vi "nanocal -- nuclear schottky fit V4.vi"() -> ()   [LabVIEW 2020] (continued)
RAW_cal__ref_"="IDS0317_210901_RAW_cal_CeCoIn5_4th_046(132)_C(f)_12T_0.43K_45deg_Tdep_raw_.dat", "IDS0317_210901_RAW_cal__sam_"="IDS0317_210901_RAW_cal_CeCoIn5_4th_046(132)_C(f)_12T_0.43K_45deg_Tdep_raw_.dat", "IDS0318_210901_RAW_cal__ref_"="IDS0318_210901_RAW_cal_CeCoIn5_4th_047(133)_C(f)_12T_0.53K_45deg_Tdep_raw_.dat", "IDS0318_210901_RAW_cal__sam_"="IDS0318_210901_RAW_cal_CeCoIn5_4th_047(133)_C(f)_12T_0.53K_45deg_Tdep_raw_.dat", "IDS0319_210901_RAW_cal__ref_"="IDS0319_210901_RAW_cal_CeCoIn5_4th_048(134)_C(f)_12T_0.62K_45deg_Tdep_raw_.dat", "IDS0319_210901_RAW_cal__sam_"="IDS0319_210901_RAW_cal_CeCoIn5_4th_048(134)_C(f)_12T_0.62K_45deg_Tdep_raw_.dat", "IDS0320_210901_RAW_cal__ref_"="IDS0320_210901_RAW_cal_CeCoIn5_4th_049(135)_C(f)_12T_0.83K_45deg_Tdep_raw_.dat", "IDS0320_210901_RAW_cal__sam_"="IDS0320_210901_RAW_cal_CeCoIn5_4th_049(135)_C(f)_12T_0.83K_45deg_Tdep_raw_.dat", "IDS0321_210901_RAW_cal__ref_"="IDS0321_210901_RAW_cal_CeCoIn5_4th_050(136)_C(f)_12T_1.13K_45deg_Tdep_raw_.dat", "IDS0321_210901_RAW_cal__sam_"="IDS0321_210901_RAW_cal_CeCoIn5_4th_050(136)_C(f)_12T_1.13K_45deg_Tdep_raw_.dat", "IDS0322_210901_RAW_cal__ref_"="IDS0322_210901_RAW_cal_CeCoIn5_4th_051(137)_C(f)_12T_1.90K_45deg_Tdep_raw_.dat", "IDS0322_210901_RAW_cal__sam_"="IDS0322_210901_RAW_cal_CeCoIn5_4th_051(137)_C(f)_12T_1.90K_45deg_Tdep_raw_.dat", "IDS0323_210901_RAW_cal__ref_"="IDS0323_210901_RAW_cal_CeCoIn5_4th_052(138)_C(f)_12T_3.10K_45deg_Tdep_raw_.dat", "IDS0323_210901_RAW_cal__sam_"="IDS0323_210901_RAW_cal_CeCoIn5_4th_052(138)_C(f)_12T_3.10K_45deg_Tdep_raw_.dat", "IDS0324_210901_RAW_cal__ref_"="IDS0324_210901_RAW_cal_CeCoIn5_4th_053(139)_C(f)_12T_5.70K_45deg_Tdep_raw_.dat", "IDS0324_210901_RAW_cal__sam_"="IDS0324_210901_RAW_cal_CeCoIn5_4th_053(139)_C(f)_12T_5.70K_45deg_Tdep_raw_.dat", "IDS0330_210901_RAW_cal__ref_"="IDS0330_210901_RAW_cal_CeCoIn5_4th_059_C(f)_1T_0.197K_90deg_Bdep_raw_.dat", "IDS0330_210901_RAW_cal__sam_"="IDS0330_210901_RAW_cal_CeCoIn5_4th_059_C(f)_1T_0.197K_90deg_Bdep_raw_.dat", "IDS0331_210901_RAW_cal__ref_"="IDS0331_210901_RAW_cal_CeCoIn5_4th_060_C(f)_2T_0.197K_90deg_Bdep_raw_.dat", "IDS0331_210901_RAW_cal__sam_"="IDS0331_210901_RAW_cal_CeCoIn5_4th_060_C(f)_2T_0.197K_90deg_Bdep_raw_.dat", "IDS0335_210904_RAW_cal__ref_"="IDS0335_210904_RAW_cal_CeCoIn5_4th_064_C(f)_5.0T_0.197K_90deg_fsweep_Tdep_raw_.dat", "IDS0335_210904_RAW_cal__sam_"="IDS0335_210904_RAW_cal_CeCoIn5_4th_064_C(f)_5.0T_0.197K_90deg_fsweep_Tdep_raw_.dat", "IDS0336_210904_RAW_cal__ref_"="IDS0336_210904_RAW_cal_CeCoIn5_4th_065_C(f)_5.0T_0.122K_90deg_fsweep_Tdep_raw_.dat", "IDS0336_210904_RAW_cal__sam_"="IDS0336_210904_RAW_cal_CeCoIn5_4th_065_C(f)_5.0T_0.122K_90deg_fsweep_Tdep_raw_.dat", "IDS0337_210904_RAW_cal__ref_"="IDS0337_210904_RAW_cal_CeCoIn5_4th_066_C(f)_5.0T_0.157K_90deg_Tdep_raw_.dat", "IDS0337_210904_RAW_cal__sam_"="IDS0337_210904_RAW_cal_CeCoIn5_4th_066_C(f)_5.0T_0.157K_90deg_Tdep_raw_.dat", "IDS0338_210904_RAW_cal__ref_"="IDS0338_210904_RAW_cal_CeCoIn5_4th_067_C(f)_5.0T_0.170K_90deg_Tdep_raw_.dat", "IDS0338_210904_RAW_cal__sam_"="IDS0338_210904_RAW_cal_CeCoIn5_4th_067_C(f)_5.0T_0.170K_90deg_Tdep_raw_.dat", "IDS0339_210904_RAW_cal__ref_"="IDS0339_210904_RAW_cal_CeCoIn5_4th_068_C(f)_5.0T_0.255K_90deg_Tdep_raw_.dat", "IDS0339_210904_RAW_cal__sam_"="IDS0339_210904_RAW_cal_CeCoIn5_4th_068_C(f)_5.0T_0.255K_90deg_Tdep_raw_.dat", "IDS0340_210904_RAW_cal__ref_"="IDS0340_210904_RAW_cal_CeCoIn5_4th_069_C(f)_5.0T_0.308K_90deg_Tdep_raw_.dat", "IDS0340_210904_RAW_cal__sam_"="IDS0340_210904_RAW_cal_CeCoIn5_4th_069_C(f)_5.0T_0.308K_90deg_Tdep_raw_.dat", "IDS0341_210904_RAW_cal__ref_"="IDS0341_210904_RAW_cal_CeCoIn5_4th_070_C(f)_5.0T_0.360K_90deg_Tdep_raw_.dat", "IDS0341_210904_RAW_cal__sam_"="IDS0341_210904_RAW_cal_CeCoIn5_4th_070_C(f)_5.0T_0.360K_90deg_Tdep_raw_.dat", "IDS0342_210904_RAW_cal__ref_"="IDS0342_210904_RAW_cal_CeCoIn5_4th_071_C(f)_5.0T_0.438K_90deg_Tdep_raw_.dat", "IDS0342_210904_RAW_cal__sam_"="IDS0342_210904_RAW_cal_CeCoIn5_4th_071_C(f)_5.0T_0.438K_90deg_Tdep_raw_.dat", "IDS0343_210904_RAW_cal__ref_"="IDS0343_210904_RAW_cal_CeCoIn5_4th_072_C(f)_5.0T_0.53K_90deg_Tdep_raw_.dat", "IDS0343_210904_RAW_cal__sam_"="IDS0343_210904_RAW_cal_CeCoIn5_4th_072_C(f)_5.0T_0.53K_90deg_Tdep_raw_.dat", "IDS0344_210904_RAW_cal__ref_"="IDS0344_210904_RAW_cal_CeCoIn5_4th_073_C(f)_5.0T_0.62K_90deg_Tdep_raw_.dat", "IDS0344_210904_RAW_cal__sam_"="IDS0344_210904_RAW_cal_CeCoIn5_4th_073_C(f)_5.0T_0.62K_90deg_Tdep_raw_.dat", "IDS0346_210904_RAW_cal__ref_"="IDS0346_210904_RAW_cal_CeCoIn5_4th_075_C(f)_8.0T_0.122K_90deg_Tdep_raw_.dat", "IDS0346_210904_RAW_cal__sam_"="IDS0346_210904_RAW_cal_CeCoIn5_4th_075_C(f)_8.0T_0.122K_90deg_Tdep_raw_.dat", "IDS0347_210906_RAW_cal__ref_"="IDS0347_210906_RAW_cal_CeCoIn5_4th_076_C(f)_8.0T_0.157K_90deg_Tdep_raw_.dat", "IDS0347_210906_RAW_cal__sam_"="IDS0347_210906_RAW_cal_CeCoIn5_4th_076_C(f)_8.0T_0.157K_90deg_Tdep_raw_.dat", "IDS0348_210906_RAW_cal__ref_"="IDS0348_210906_RAW_cal_CeCoIn5_4th_077_C(f)_8.0T_0.178K_90deg_Tdep_raw_.dat", "IDS0348_210906_RAW_cal__sam_"="IDS0348_210906_RAW_cal_CeCoIn5_4th_077_C(f)_8.0T_0.178K_90deg_Tdep_raw_.dat", "IDS0349_210906_RAW_cal__ref_"="IDS0349_210906_RAW_cal_CeCoIn5_4th_078_C(f)_8.0T_0.20K_90deg_Tdep_raw_.dat", "IDS0349_210906_RAW_cal__sam_"="IDS0349_210906_RAW_cal_CeCoIn5_4th_078_C(f)_8.0T_0.20K_90deg_Tdep_raw_.dat", "IDS0350_210906_RAW_cal__ref_"="IDS0350_210906_RAW_cal_CeCoIn5_4th_079_C(f)_8.0T_0.26K_90deg_Tdep_raw_.dat", "IDS0350_210906_RAW_cal__sam_"="IDS0350_210906_RAW_cal_CeCoIn5_4th_079_C(f)_8.0T_0.26K_90deg_Tdep_raw_.dat", "IDS0351_210906_RAW_cal__ref_"="IDS0351_210906_RAW_cal_CeCoIn5_4th_080_C(f)_8.0T_0.31K_90deg_Tdep_raw_.dat", "IDS0351_210906_RAW_cal__sam_"="IDS0351_210906_RAW_cal_CeCoIn5_4th_080_C(f)_8.0T_0.31K_90deg_Tdep_raw_.dat", "IDS0352_210906_RAW_cal__ref_"="IDS0352_210906_RAW_cal_CeCoIn5_4th_081_C(f)_8.0T_0.36K_90deg_Tdep_raw_.dat", "IDS0352_210906_RAW_cal__sam_"="IDS0352_210906_RAW_cal_CeCoIn5_4th_081_C(f)_8.0T_0.36K_90deg_Tdep_raw_.dat", "IDS0353_210906_RAW_cal__ref_"="IDS0353_210906_RAW_cal_CeCoIn5_4th_082_C(f)_8.0T_0.438K_90deg_Tdep_raw_.dat", "IDS0353_210906_RAW_cal__sam_"="IDS0353_210906_RAW_cal_CeCoIn5_4th_082_C(f)_8.0T_0.438K_90deg_Tdep_raw_.dat", "IDS0354_210906_RAW_cal__ref_"="IDS0354_210906_RAW_cal_CeCoIn5_4th_083_C(f)_8.0T_0.53K_90deg_Tdep_raw_.dat", "IDS0354_210906_RAW_cal__sam_"="IDS0354_210906_RAW_cal_CeCoIn5_4th_083_C(f)_8.0T_0.53K_90deg_Tdep_raw_.dat", "IDS0355_210906_RAW_cal__ref_"="IDS0355_210906_RAW_cal_CeCoIn5_4th_085_C(f)_8.0T_0.83K_90deg_Tdep_raw_.dat", "IDS0355_210906_RAW_cal__sam_"="IDS0355_210906_RAW_cal_CeCoIn5_4th_085_C(f)_8.0T_0.83K_90deg_Tdep_raw_.dat", "IDS0359_210907_RAW_cal__ref_"="IDS0359_210907_RAW_cal_CeCoIn5_4th_089_C(f)_12.0T_0.12K_60deg_Tdep_raw_.dat", "IDS0359_210907_RAW_cal__sam_"="IDS0359_210907_RAW_cal_CeCoIn5_4th_089_C(f)_12.0T_0.12K_60deg_Tdep_raw_.dat", "IDS0360_210907_RAW_cal__ref_"="IDS0360_210907_RAW_cal_CeCoIn5_4th_090_C(f)_12.0T_0.15K_60deg_Tdep_raw_.dat", "IDS0360_210907_RAW_cal__sam_"="IDS0360_210907_RAW_cal_CeCoIn5_4th_090_C(f)_12.0T_0.15K_60deg_Tdep_raw_.dat", "IDS0361_210908_RAW_cal__ref_"="IDS0361_210908_RAW_cal_CeCoIn5_4th_091_C(f)_12.0T_0.168K_60deg_Tdep_raw_.dat", "IDS0361_210908_RAW_cal__sam_"="IDS0361_210908_RAW_cal_CeCoIn5_4th_091_C(f)_12.0T_0.168K_60deg_Tdep_raw_.dat", "IDS0362_210908_RAW_cal__ref_"="IDS0362_210908_RAW_cal_CeCoIn5_4th_092_C(f)_12.0T_0.197K_60deg_Tdep_raw_.dat", "IDS0362_210908_RAW_cal__sam_"="IDS0362_210908_RAW_cal_CeCoIn5_4th_092_C(f)_12.0T_0.197K_60deg_Tdep_raw_.dat", "IDS0363_210908_RAW_cal__ref_"="IDS0363_210908_RAW_cal_CeCoIn5_4th_093_C(f)_12.0T_0.25K_60deg_Tdep_raw_.dat", "IDS0363_210908_RAW_cal__sam_"="IDS0363_210908_RAW_cal_CeCoIn5_4th_093_C(f)_12.0T_0.25K_60deg_Tdep_raw_.dat", "IDS0364_210908_RAW_cal__ref_"="IDS0364_210908_RAW_cal_CeCoIn5_4th_094_C(f)_12.0T_0.307K_60deg_Tdep_raw_.dat", "IDS0364_210908_RAW_cal__sam_"="IDS0364_210908_RAW_cal_CeCoIn5_4th_094_C(f)_12.0T_0.307K_60deg_Tdep_raw_.dat", "IDS0365_210908_RAW_cal__ref_"="IDS0365_210908_RAW_cal_CeCoIn5_4th_095_C(f)_12.0T_0.36K_60deg_Tdep_raw_.dat", "IDS0365_210908_RAW_cal__sam_"="IDS0365_210908_RAW_cal_CeCoIn5_4th_095_C(f)_12.0T_0.36K_60deg_Tdep_raw_.dat", "IDS0366_210908_RAW_cal__ref_"="IDS0366_210908_RAW_cal_CeCoIn5_4th_096_C(f)_12.0T_0.43K_60deg_Tdep_raw_.dat", "IDS0366_210908_RAW_cal__sam_"="IDS0366_210908_RAW_cal_CeCoIn5_4th_096_C(f)_12.0T_0.43K_60deg_Tdep_raw_.dat", "IDS0367_210908_RAW_cal__ref_"="IDS0367_210908_RAW_cal_CeCoIn5_4th_097_C(f)_12.0T_0.53K_60deg_Tdep_raw_.dat", "IDS0367_210908_RAW_cal__sam_"="IDS0367_210908_RAW_cal_CeCoIn5_4th_097_C(f)_12.0T_0.53K_60deg_Tdep_raw_.dat", "IDS0368_210908_RAW_cal__ref_"="IDS0368_210908_RAW_cal_CeCoIn5_4th_098_C(f)_12.0T_0.63K_60deg_Tdep_raw_.dat", "IDS0368_210908_RAW_cal__sam_"="IDS0368_210908_RAW_cal_CeCoIn5_4th_098_C(f)_12.0T_0.63K_60deg_Tdep_raw_.dat", "IDS0369_210908_RAW_cal__ref_"="IDS0369_210908_RAW_cal_CeCoIn5_4th_099_C(f)_12.0T_0.83K_60deg_Tdep_raw_.dat", "IDS0369_210908_RAW_cal__sam_"="IDS0369_210908_RAW_cal_CeCoIn5_4th_099_C(f)_12.0T_0.83K_60deg_Tdep_raw_.dat", "IDS0370_210908_RAW_cal__ref_"="IDS0370_210908_RAW_cal_CeCoIn5_4th_100_C(f)_12.0T_1.13K_60deg_Tdep_raw_.dat", "IDS0370_210908_RAW_cal__sam_"="IDS0370_210908_RAW_cal_CeCoIn5_4th_100_C(f)_12.0T_1.13K_60deg_Tdep_raw_.dat", "IDS0371_210908_RAW_cal__ref_"="IDS0371_210908_RAW_cal_CeCoIn5_4th_101_C(f)_12.0T_1.90K_60deg_Tdep_raw_.dat", "IDS0371_210908_RAW_cal__sam_"="IDS0371_210908_RAW_cal_CeCoIn5_4th_101_C(f)_12.0T_1.90K_60deg_Tdep_raw_.dat", "IDS0372_210908_RAW_cal__ref_"="IDS0372_210908_RAW_cal_CeCoIn5_4th_102_C(f)_12.0T_3.11K_60deg_Tdep_raw_.dat", "IDS0372_210908_RAW_cal__sam_"="IDS0372_210908_RAW_cal_CeCoIn5_4th_102_C(f)_12.0T_3.11K_60deg_Tdep_raw_.dat", "IDS0373_210908_RAW_cal__ref_"="IDS0373_210908_RAW_cal_CeCoIn5_4th_103_C(f)_12.0T_5.75K_60deg_Tdep_raw_.dat", "IDS0373_210908_RAW_cal__sam_"="IDS0373_210908_RAW_cal_CeCoIn5_4th_103_C(f)_12.0T_5.75K_60deg_Tdep_raw_.dat", "IDS0377_210909_RAW_cal__ref_"="IDS0377_210909_RAW_cal_CeCoIn5_4th_107_C(f)_8.0T_0.197K_0deg_Tdep_raw_.dat", "IDS0377_210909_RAW_cal__sam_"="IDS0377_210909_RAW_cal_CeCoIn5_4th_107_C(f)_8.0T_0.197K_0deg_Tdep_raw_.dat", "IDS0378_210909_RAW_cal__ref_"="IDS0378_210909_RAW_cal_CeCoIn5_4th_108_C(f)_8.0T_0.122K_0deg_Tdep_raw_.dat", "IDS0378_210909_RAW_cal__sam_"="IDS0378_210909_RAW_cal_CeCoIn5_4th_108_C(f)_8.0T_0.122K_0deg_Tdep_raw_.dat", "IDS0379_210909_RAW_cal__ref_"="IDS0379_210909_RAW_cal_CeCoIn5_4th_109_C(f)_8.0T_0.148K_0deg_Tdep_raw_.dat", "IDS0379_210909_RAW_cal__sam_"="IDS0379_210909_RAW_cal_CeCoIn5_4th_109_C(f)_8.0T_0.148K_0deg_Tdep_raw_.dat", "IDS0380_210909_RAW_cal__ref_"="IDS0380_210909_RAW_cal_CeCoIn5_4th_110_C(f)_8.0T_0.168K_0deg_Tdep_raw_.dat", "IDS0380_210909_RAW_cal__sam_"="IDS0380_210909_RAW_cal_CeCoIn5_4th_110_C(f)_8.0T_0.168K_0deg_Tdep_raw_.dat", "IDS0381_210909_RAW_cal__ref_"="IDS0381_210909_RAW_cal_CeCoIn5_4th_111_C(f)_8.0T_0.25K_0deg_Tdep_raw_.dat", "IDS0381_210909_RAW_cal__sam_"="IDS0381_210909_RAW_cal_CeCoIn5_4th_111_C(f)_8.0T_0.25K_0deg_Tdep_raw_.dat", "IDS0382_210909_RAW_cal__ref_"="IDS0382_210909_RAW_cal_CeCoIn5_4th_112_C(f)_8.0T_0.30K_0deg_Tdep_raw_.dat", "IDS0382_210909_RAW_cal__sam_"="IDS0382_210909_RAW_cal_CeCoIn5_4th_112_C(f)_8.0T_0.30K_0deg_Tdep_raw_.dat", "IDS0383_210910_RAW_cal__ref_"="IDS0383_210910_RAW_cal_CeCoIn5_4th_113_C(f)_8.0T_0.36K_0deg_Tdep_raw_.dat", "IDS0383_210910_RAW_cal__sam_"="IDS0383_210910_RAW_cal_CeCoIn5_4th_113_C(f)_8.0T_0.36K_0deg_Tdep_raw_.dat", "IDS0384_210910_RAW_cal__ref_"="IDS0384_210910_RAW_cal_CeCoIn5_4th_114_C(f)_8.0T_0.43K_0deg_Tdep_raw_.dat", "IDS0384_210910_RAW_cal__sam_"="IDS0384_210910_RAW_cal_CeCoIn5_4th_114_C(f)_8.0T_0.43K_0deg_Tdep_raw_.dat", "IDS0385_210910_RAW_cal__ref_"="IDS0385_210910_RAW_cal_CeCoIn5_4th_115_C(f)_8.0T_0.53K_0deg_Tdep_raw_.dat", "IDS0385_210910_RAW_cal__sam_"="IDS0385_210910_RAW_cal_CeCoIn5_4th_115_C(f)_8.0T_0.53K_0deg_Tdep_raw_.dat", "IDS0386_210910_RAW_cal__ref_"="IDS0386_210910_RAW_cal_CeCoIn5_4th_116_C(f)_8.0T_0.63K_0deg_Tdep_raw_.dat", "IDS0386_210910_RAW_cal__sam_"="IDS0386_210910_RAW_cal_CeCoIn5_4th_116_C(f)_8.0T_0.63K_0deg_Tdep_raw_.dat", "IDS0387_210910_RAW_cal__ref_"="IDS0387_210910_RAW_cal_CeCoIn5_4th_117_C(f)_8.0T_0.83K_0deg_Tdep_raw_.dat", "IDS0387_210910_RAW_cal__sam_"="IDS0387_210910_RAW_cal_CeCoIn5_4th_117_C(f)_8.0T_0.83K_0deg_Tdep_raw_.dat", "IDS0388_210910_RAW_cal__ref_"="IDS0388_210910_RAW_cal_CeCoIn5_4th_118_C(f)_8.0T_1.13K_0deg_Tdep_raw_.dat", "IDS0388_210910_RAW_cal__sam_"="IDS0388_210910_RAW_cal_CeCoIn5_4th_118_C(f)_8.0T_1.13K_0deg_Tdep_raw_.dat", "IDS0389_210910_RAW_cal__ref_"="IDS0389_210910_RAW_cal_CeCoIn5_4th_119_C(f)_8.0T_1.52K_0deg_Tdep_raw_.dat", "IDS0389_210910_RAW_cal__sam_"="IDS0389_210910_RAW_cal_CeCoIn5_4th_119_C(f)_8.0T_1.52K_0deg_Tdep_raw_.dat", "IDS0390_210910_RAW_cal__ref_"="IDS0390_210910_RAW_cal_CeCoIn5_4th_120_C(f)_8.0T_1.90K_0deg_Tdep_raw_.dat", "IDS0390_210910_RAW_cal__sam_"="IDS0390_210910_RAW_cal_CeCoIn5_4th_120_C(f)_8.0T_1.90K_0deg_Tdep_raw_.dat", "IDS0391_210910_RAW_cal__ref_"="IDS0391_210910_RAW_cal_CeCoIn5_4th_121_C(f)_8.0T_1.25K_0deg_Tdep_raw_.dat", "IDS0391_210910_RAW_cal__sam_"="IDS0391_210910_RAW_cal_CeCoIn5_4th_121_C(f)_8.0T_1.25K_0deg_Tdep_raw_.dat", "IDS0392_210910_RAW_cal__ref_"="IDS0392_210910_RAW_cal_CeCoIn5_4th_122_C(f)_8.0T_1.39K_0deg_Tdep_raw_.dat", "IDS0392_210910_RAW_cal__sam_"="IDS0392_210910_RAW_cal_CeCoIn5_4th_122_C(f)_8.0T_1.39K_0deg_Tdep_raw_.dat", "IDS0393_210910_RAW_cal__ref_"="IDS0393_210910_RAW_cal_CeCoIn5_4th_123_C(f)_8.0T_3.11K_0deg_Tdep_raw_.dat", "IDS0393_210910_RAW_cal__sam_"="IDS0393_210910_RAW_cal_CeCoIn5_4th_123_C(f)_8.0T_3.11K_0deg_Tdep_raw_.dat", "IDS0394_210910_RAW_cal__ref_"="IDS0394_210910_RAW_cal_CeCoIn5_4th_124_C(f)_8.0T_5.75K_0deg_Tdep_raw_.dat", "IDS0394_210910_RAW_cal__sam_"="IDS0394_210910_RAW_cal_CeCoIn5_4th_124_C(f)_8.0T_5.75K_0deg_Tdep_raw_.dat", "IDS0395_210910_RAW_cal__ref_"="IDS0395_210910_RAW_cal_CeCoIn5_4th_125_C(f)_8.0T_1.31K_0deg_Tdep_raw_.dat", "IDS0395_210910_RAW_cal__sam_"="IDS0395_210910_RAW_cal_CeCoIn5_4th_125_C(f)_8.0T_1.31K_0deg_Tdep_raw_.dat"}
  out "temps&degs":map{string, map{T5, dbl}}(c390)
  out "mathematica thing":map{string, map{T5, dbl}}(c390)
  out "constrained filename lookup":map{i32, string}(c390)={0="IDS0378_210909_RAW_cal__ref_", 1="IDS0379_210909_RAW_cal__ref_", 2="IDS0380_210909_RAW_cal__ref_", 3="IDS0377_210909_RAW_cal__ref_", 4="IDS0381_210909_RAW_cal__ref_", 5="IDS0382_210909_RAW_cal__ref_", 6="IDS0383_210910_RAW_cal__ref_", 7="IDS0384_210910_RAW_cal__ref_", 8="IDS0385_210910_RAW_cal__ref_", 9="IDS0386_210910_RAW_cal__ref_", 10="IDS0387_210910_RAW_cal__ref_", 11="IDS0388_210910_RAW_cal__ref_", 12="IDS0391_210910_RAW_cal__ref_", 13="IDS0395_210910_RAW_cal__ref_", 14="IDS0392_210910_RAW_cal__ref_", 15="IDS0389_210910_RAW_cal__ref_", 16="IDS0390_210910_RAW_cal__ref_", 17="IDS0393_210910_RAW_cal__ref_", 18="IDS0394_210910_RAW_cal__ref_"}
  out "filesnames lookup":map{i32, string}(c390)={0="IDS0183_210310_RAW_cal__sam_", 1="IDS0311_210901_RAW_cal__sam_", 2="IDS0359_210907_RAW_cal__sam_", 3="IDS0336_210904_RAW_cal__sam_", 4="IDS0346_210904_RAW_cal__sam_", 5="IDS0378_210909_RAW_cal__sam_", 6="IDS0158_210310_RAW_cal__sam_", 7="IDS0300_210427_RAW_cal__sam_", 8="IDS0184_210310_RAW_cal__sam_", 9="IDS0210_210310_RAW_cal__sam_", 10="IDS0379_210909_RAW_cal__sam_", 11="IDS0360_210907_RAW_cal__sam_", 12="IDS0310_210901_RAW_cal__sam_", 13="IDS0337_210904_RAW_cal__sam_", 14="IDS0347_210906_RAW_cal__sam_", 15="IDS0305_210831_RAW_cal__sam_", 16="IDS0361_210908_RAW_cal__sam_", 17="IDS0380_210909_RAW_cal__sam_", 18="IDS0159_210310_RAW_cal__sam_", 19="IDS0304_210831_RAW_cal__sam_", 20="IDS0312_210901_RAW_cal__sam_", 21="IDS0338_210904_RAW_cal__sam_", 22="IDS0348_210906_RAW_cal__sam_", 23="IDS0181_210310_RAW_cal__sam_", 24="IDS0185_210310_RAW_cal__sam_", 25="IDS0208_210310_RAW_cal__sam_", 26="IDS0209_210310_RAW_cal__sam_", 27="IDS0211_210310_RAW_cal__sam_", 28="IDS0212_210310_RAW_cal__sam_", 29="IDS0213_210310_RAW_cal__sam_", 30="IDS0214_210310_RAW_cal__sam_", 31="IDS0215_210310_RAW_cal__sam_", 32="IDS0216_210310_RAW_cal__sam_", 33="IDS0217_210310_RAW_cal__sam_", 34="IDS0330_210901_RAW_cal__sam_", 35="IDS0331_210901_RAW_cal__sam_", 36="IDS0335_210904_RAW_cal__sam_", 37="IDS0362_210908_RAW_cal__sam_", 38="IDS0377_210909_RAW_cal__sam_", 39="IDS0160_210310_RAW_cal__sam_", 40="IDS0303_210831_RAW_cal__sam_", 41="IDS0313_210901_RAW_cal__sam_", 42="IDS0349_210906_RAW_cal__sam_", 43="IDS0161_210310_RAW_cal__sam_", 44="IDS0186_210310_RAW_cal__sam_", 45="IDS0302_210831_RAW_cal__sam_", 46="IDS0363_210908_RAW_cal__sam_", 47="IDS0381_210909_RAW_cal__sam_", 48="IDS0314_210901_RAW_cal__sam_", 49="IDS0339_210904_RAW_cal__sam_", 50="IDS0350_210906_RAW_cal__sam_", 51="IDS0162_210310_RAW_cal__sam_", 52="IDS0187_210310_RAW_cal__sam_", 53="IDS0301_210831_RAW_cal__sam_", 54="IDS0315_210901_RAW_cal__sam_", 55="IDS0382_210909_RAW_cal__sam_", 56="IDS0364_210908_RAW_cal__sam_", 57="IDS0340_210904_RAW_cal__sam_", 58="IDS0351_210906_RAW_cal__sam_", 59="IDS0163_210310_RAW_cal__sam_", 60="IDS0188_210310_RAW_cal__sam_", 61="IDS0299_210427_RAW_cal__sam_", 62="IDS0316_210901_RAW_cal__sam_", 63="IDS0341_210904_RAW_cal__sam_", 64="IDS0352_210906_RAW_cal__sam_", 65="IDS0365_210908_RAW_cal__sam_", 66="IDS0383_210910_RAW_cal__sam_", 67="IDS0164_210310_RAW_cal__sam_", 68="IDS0189_210310_RAW_cal__sam_", 69="IDS0298_210427_RAW_cal__sam_", 70="IDS0317_210901_RAW_cal__sam_", 71="IDS0366_210908_RAW_cal__sam_", 72="IDS0384_210910_RAW_cal__sam_", 73="IDS0342_210904_RAW_cal__sam_", 74="IDS0353_210906_RAW_cal__sam_", 75="IDS0165_210310_RAW_cal__sam_", 76="IDS0190_210310_RAW_cal__sam_", 77="IDS0297_210427_RAW_cal__sam_", 78="IDS0318_210901_RAW_cal__sam_", 79="IDS0343_210904_RAW_cal__sam_", 80="IDS0354_210906_RAW_cal__sam_", 81="IDS0367_210908_RAW_cal__sam_", 82="IDS0385_210910_RAW_cal__sam_", 83="IDS0166_210310_RAW_cal__sam_", 84="IDS0191_210310_RAW_cal__sam_", 85="IDS0296_210427_RAW_cal__sam_", 86="IDS0319_210901_RAW_cal__sam_", 87="IDS0344_210904_RAW_cal__sam_", 88="IDS0368_210908_RAW_cal__sam_", 89="IDS0386_210910_RAW_cal__sam_", 90="IDS0220_210310_RAW_cal__sam_", 91="IDS0167_210310_RAW_cal__sam_", 92="IDS0192_210310_RAW_cal__sam_", 93="IDS0295_210427_RAW_cal__sam_", 94="IDS0320_210901_RAW_cal__sam_", 95="IDS0355_210906_RAW_cal__sam_", 96="IDS0369_210908_RAW_cal__sam_", 97="IDS0387_210910_RAW_cal__sam_", 98="IDS0168_210310_RAW_cal__sam_", 99="IDS0219_210310_RAW_cal__sam_", 100="IDS0193_210310_RAW_cal__sam_", 101="IDS0294_210427_RAW_cal__sam_", 102="IDS0321_210901_RAW_cal__sam_", 103="IDS0370_210908_RAW_cal__sam_", 104="IDS0388_210910_RAW_cal__sam_", 105="IDS0169_210310_RAW_cal__sam_", 106="IDS0391_210910_RAW_cal__sam_", 107="IDS0395_210910_RAW_cal__sam_", 108="IDS0392_210910_RAW_cal__sam_", 109="IDS0389_210910_RAW_cal__sam_", 110="IDS0218_210310_RAW_cal__sam_", 111="IDS0194_210310_RAW_cal__sam_", 112="IDS0293_210427_RAW_cal__sam_", 113="IDS0322_210901_RAW_cal__sam_", 114="IDS0371_210908_RAW_cal__sam_", 115="IDS0390_210910_RAW_cal__sam_", 116="IDS0170_210310_RAW_cal__sam_", 117="IDS0195_210310_RAW_cal__sam_", 118="IDS0306_210831_RAW_cal__sam_", 119="IDS0323_210901_RAW_cal__sam_", 120="IDS0372_210908_RAW_cal__sam_", 121="IDS0393_210910_RAW_cal__sam_", 122="IDS0171_210310_RAW_cal__sam_", 123="IDS0196_210310_RAW_cal__sam_", 124="IDS0324_210901_RAW_cal__sam_", 125="IDS0373_210908_RAW_cal__sam_", 126="IDS0394_210910_RAW_cal__sam_", 127="IDS0172_210310_RAW_cal__sam_"}
  out "Set of B's":set{dbl}(c389)={0.0, 1.0, 2.0, 5.0, 6.0, 7.0, 8.0, 9.0, 10.0, 11.0, 12.0}
  out "Set of θ's":set{dbl}(c389)={0.0, 30.0, 45.0, 60.0, 90.0}
  out "Set of T's":set{dbl}(c389)={0.12, 0.122, 0.14, 0.148, 0.15, 0.157, 0.16, 0.168, 0.17, 0.178, 0.179, 0.197, 0.2, 0.22, 0.249, 0.25, 0.255, 0.26, 0.28, 0.3, 0.307, 0.308, 0.31, 0.33, 0.36, 0.4, 0.43, 0.438, 0.48, 0.512, 0.53, 0.58, 0.61, 0.62, 0.63, 0.677, 0.68, 0.81, 0.83, 0.91, 1.0, 1.1, 1.13, 1.23, 1.25, 1.31, 1.39, 1.52, 1.55, 1.8, 1.9, 1.97, 3.0, 3.1, 3.11, 3.19, 5.7, 5.75, 5.8}
  out "B lookup":map{i32, dbl}(c390)={0=0.0, 1=1.0, 2=2.0, 3=5.0, 4=6.0, 5=7.0, 6=8.0, 7=9.0, 8=10.0, 9=11.0, 10=12.0}
  out "θ lookup":map{i32, dbl}(c390)={0=0.0, 1=30.0, 2=45.0, 3=60.0, 4=90.0}
  out "T lookup":map{i32, dbl}(c390)={0=0.12, 1=0.122, 2=0.14, 3=0.148, 4=0.15, 5=0.157, 6=0.16, 7=0.168, 8=0.17, 9=0.178, 10=0.179, 11=0.197, 12=0.2, 13=0.22, 14=0.249, 15=0.25, 16=0.255, 17=0.26, 18=0.28, 19=0.3, 20=0.307, 21=0.308, 22=0.31, 23=0.33, 24=0.36, 25=0.4, 26=0.43, 27=0.438, 28=0.48, 29=0.512, 30=0.53, 31=0.58, 32=0.61, 33=0.62, 34=0.63, 35=0.677, 36=0.68, 37=0.81, 38=0.83, 39=0.91, 40=1.0, 41=1.1, 42=1.13, 43=1.23, 44=1.25, 45=1.31, 46=1.39, 47=1.52, 48=1.55, 49=1.8, 50=1.9, 51=1.97, 52=3.0, 53=3.1, 54=3.11, 55=3.19, 56=5.7, 57=5.75, 58=5.8}
  out "Set of Change":set{dbl}(c389)={1.0, 2.0}
  out "change lookup":map{i32, dbl}(c390)={0=1.0, 1=2.0}
  out "side map from NUM":map{i32, T14}(c390)={4000=enum."ref", 8000=enum."sam"}
  out "side map to STR":map{T14, string}(c390)={enum."sam"="_sam_", enum."ref"="_ref_"}
  out "side map to NUM":map{T14, i32}(c390)={enum."sam"=8000, enum."ref"=4000}
  out "data file parameters map":map{T5, T15}(c390)={enum."T (K)"=enum."get T", enum."B (T)"=enum."get B", enum."θ (deg)"=enum."get deg", enum."change (B|T)"=enum."get change"}
  out "Side lookup":map{i32, dbl}(c390)={0=4000.0, 1=8000.0}
  out "Set of Sides":set{dbl}(c389)={4000.0, 8000.0}
  in  "backup string :b":string=" <| \"ζ\"->  0.167234158379  , \"τ1\"-> 0.020665214756  , \"τS\"-> 0.072250691270  , \"τN\"-> 0.020708769022  , \"τC\"-> 0.001243822553  , \"κ0\"-> 0.000000001059  , \"mm1\"-> 0.000000000000  , \"mm2\"-> 0.000000000000  , \"mm3\"-> 0.000000000000  , \"T\"->  5.700000000000  , \"B\"-> 12.000000000000  , \"θ\"-> 45.000000000000  |> "
  in  "tab 7":enum32{"Page 1"}(tab)
  in  "tab 3":enum32{"Page 1"}(tab)
  out "key":string="IDS0340_210904_RAW_cal__ref_"
  out "T (K)":dbl=0.308 format="%#_10f"
  out "θ (deg)":dbl=90.0 format="%#_10f"
  out "B (T)":dbl=5.0
  in  "tab 6":enum32{"Page 1"}(tab)
  in  "write τ to Math! :p":bool
  in  "constrained filenames :|\\":u16(ring)=5 caption="files" items=["IDS0378_210909_RAW_cal_CeCoIn5_4th_108_C(f)_8.0T_0.122K_0deg_Tdep_raw_.dat", "IDS0379_210909_RAW_cal_CeCoIn5_4th_109_C(f)_8.0T_0.148K_0deg_Tdep_raw_.dat", "IDS0380_210909_RAW_cal_CeCoIn5_4th_110_C(f)_8.0T_0.168K_0deg_Tdep_raw_.dat", "IDS0377_210909_RAW_cal_CeCoIn5_4th_107_C(f)_8.0T_0.197K_0deg_Tdep_raw_.dat", "IDS0381_210909_RAW_cal_CeCoIn5_4th_111_C(f)_8.0T_0.25K_0deg_Tdep_raw_.dat", "IDS0382_210909_RAW_cal_CeCoIn5_4th_112_C(f)_8.0T_0.30K_0deg_Tdep_raw_.dat", "IDS0383_210910_RAW_cal_CeCoIn5_4th_113_C(f)_8.0T_0.36K_0deg_Tdep_raw_.dat", "IDS0384_210910_RAW_cal_CeCoIn5_4th_114_C(f)_8.0T_0.43K_0deg_Tdep_raw_.dat", "IDS0385_210910_RAW_cal_CeCoIn5_4th_115_C(f)_8.0T_0.53K_0deg_Tdep_raw_.dat", "IDS0386_210910_RAW_cal_CeCoIn5_4th_116_C(f)_8.0T_0.63K_0deg_Tdep_raw_.dat", "IDS0387_210910_RAW_cal_CeCoIn5_4th_117_C(f)_8.0T_0.83K_0deg_Tdep_raw_.dat", "IDS0388_210910_RAW_cal_CeCoIn5_4th_118_C(f)_8.0T_1.13K_0deg_Tdep_raw_.dat", "IDS0391_210910_RAW_cal_CeCoIn5_4th_121_C(f)_8.0T_1.25K_0deg_Tdep_raw_.dat", "IDS0395_210910_RAW_cal_CeCoIn5_4th_125_C(f)_8.0T_1.31K_0deg_Tdep_raw_.dat", "IDS0392_210910_RAW_cal_CeCoIn5_4th_122_C(f)_8.0T_1.39K_0deg_Tdep_raw_.dat", "IDS0389_210910_RAW_cal_CeCoIn5_4th_119_C(f)_8.0T_1.52K_0deg_Tdep_raw_.dat", "IDS0390_210910_RAW_cal_CeCoIn5_4th_120_C(f)_8.0T_1.90K_0deg_Tdep_raw_.dat", "IDS0393_210910_RAW_cal_CeCoIn5_4th_123_C(f)_8.0T_3.11K_0deg_Tdep_raw_.dat", "IDS0394_210910_RAW_cal_CeCoIn5_4th_124_C(f)_8.0T_5.75K_0deg_Tdep_raw_.dat"]
  in  "parameter selectors":enum32{"Page 1"}(tab)
  in  "select B (T)":u16(ring)=6 items=["0.000", "1.000", "2.000", "5.000", "6.000", "7.000", "8.000", "9.000", "10.000", "11.000", "12.000"]
  in  "select θ (deg)":u16(ring) items=["0.000", "30.000", "45.000", "60.000", "90.000"]
  in  "ignore T !":bool=TRUE
  in  "select T (K)":u16(ring)=10 items=["0.120", "0.122", "0.140", "0.148", "0.150", "0.157", "0.160", "0.168", "0.170", "0.178", "0.179", "0.197", "0.200", "0.220", "0.249", "0.250", "0.255", "0.260", "0.280", "0.300", "0.307", "0.308", "0.310", "0.330", "0.360", "0.400", "0.430", "0.438", "0.480", "0.512", "0.530", "0.580", "0.610", "0.620", "0.630", "0.677", "0.680", "0.810", "0.830", "0.910", "1.000", "1.100", "1.130", "1.230", "1.250", "1.310", "1.390", "1.520", "1.550", "1.800", "1.900", "1.970", "3.000", "3.100", "3.110", "3.190", "5.700", "5.750", "5.800"]
  in  "ignore B !":bool
  in  "ignore θ !":bool
  in  "X selector":T5=enum."T (K)"
  in  "select side (8S|4R)":i32(ring) items=["4000", "8000"]
  in  "ignore side !":bool
  in  "select set (1T|2B)":i32(ring) items=["1", "2"]
  in  "ignore change !":bool
  in  "parameter selectors 2":enum32{"Page 1"}(tab)
  in  "colors":u32[](array[colorbox])=[7893503, 56538, 2062078, 16740827, 16755712, 11121611, 8285330, 9272482, 9204890]
  in  "parameter":T5[](array[typedef])=[enum."ζ", enum."τ1", enum."τS", enum."τN", enum."τC", enum."κ0"]
  in  "tab 5":enum32{"Page 1"}(tab)
  in  "read τ from Math ! :q":bool
  out "file IDS":string="IDS0340_210904_RAW_cal_"
  in  "ω0 (rad/sec)":dbl(slide)=19.063235402868393 scale=0.001..50000.0 scale format="%#_2p"
  in  "offset Re\noffset Im":cluster{"Numeric":dbl, "Numeric":dbl}(slide)={"Numeric"=-54227722.77227723, "Numeric"=0.0} scale=-1000000.0..500000.0 scale format="%#_1p"
  in  "landscape plots":enum32{"Page 1", "Page 2"}(tab)
  in  "range one":dbl(slide)=0.006965 min=0.0 max=0.3 step=1e-06 scale=0.0001..1.0 scale format="%#_3p"
  in  "one":T5=enum."τS"
  out "Plot: goodness vs parameter":cluster{"Freq out (Hz)":dbl[], dbl[]}[](graph)
  in  "plot landscape!":bool
  in  "range two":dbl(slide)=0.0039049999999999996 min=0.0 max=0.3 step=1e-06 scale=0.0001..1.0 scale format="%#_3p"
  in  "two":T5=enum."τ1"
  in  "what":enum16{"1d plots", "2d plots "}(ring)
  in  "# points":i32=200
  in  "Array":T5[](array[typedef])=[enum."ζ", enum."τ1", enum."τS", enum."τN", enum."τC"]
  in  "color Map":map{T5, u32}(c390)={enum."ζ"=7893503, enum."τ1"=56538, enum."τS"=2062078, enum."τN"=16740827, enum."τC"=16755712, enum."κ0"=11121611}
